vi "Set IO Read State Call Back.vi"(8 "error in (no error)":errorcluster, 10 "callback":cluster{}, 11 "ppara":u32) -> (0 "error out":errorcluster, 3 "ppara out":u32)   [LabVIEW 2021, in "vmmsolib.lvlib"]
doc: "DLL_API void WINAPI SetIOReadStateCallBack(void* ppara, IOReadStateCallBack callback);"
uses:
  vmmsolib.lvlib
  vmmso.dll
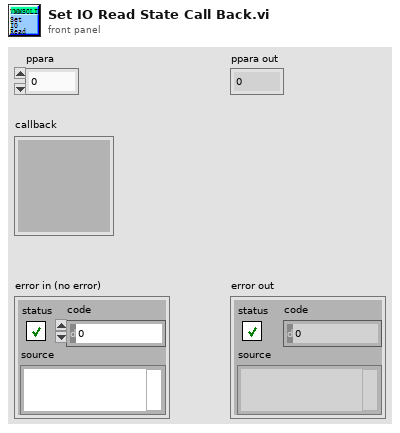
[diagram p1: front panel]
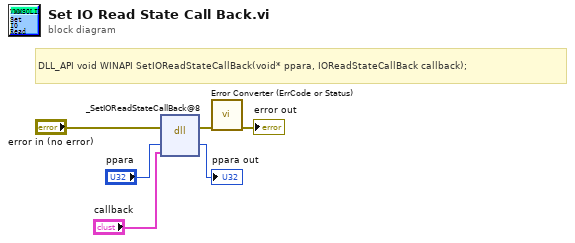
[diagram p0: block diagram]
diagram:
  # "DLL_API void WINAPI SetIOReadStateCallBack(void* ppara, IOReadStateCallBack callback);"
  n1 = dll-call lib="D:/VmMsoSDK/demo-Labview/2021/vmmsolib/vmmso.*" fn="_SetIOReadStateCallBack@8"(error in="error in (no error)", "ppara"="ppara", "callback"="callback") -> (error out=w2:errorcluster, "ppara"=→"ppara out":u32)  [unwired: 4 in, 1 out]
  n2 = call "Error Converter (ErrCode or Status).vi"("error in (no error)"=w2) -> ("error out"=→"error out":errorcluster)  [unwired: 10 in]
